vi "Answer.vi"(10 "Accident Number":i32, 11 "NxN":i32) -> (3 "Map":i32[][](array[numeric]))   [LabVIEW 2015]
panel:
  # "地圖"
  # "輸入地圖尺寸"
  # "狀況數量"
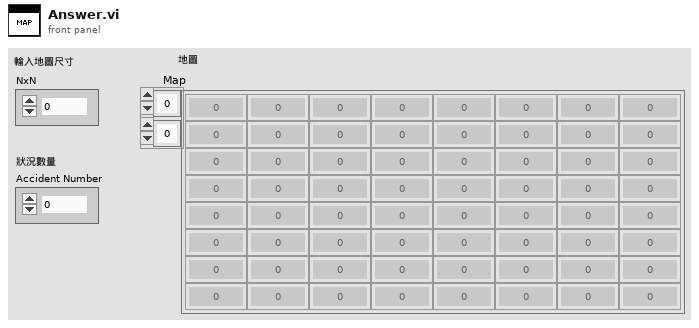
[diagram p1: front panel]
types:
  T1 = typedef "Accident Position.ctl" = cluster{"row":i32, "col":i32}
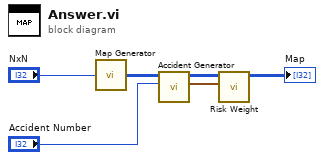
[diagram p0: block diagram]
diagram:
  n1 = call "Map Generator.vi"("NxN"="NxN") -> ("Map"=w5:i32[][])
  n2 = call "Accident Generator.vi"("Accident Number"="Accident Number", "Map"=w5) -> ("Accident Position"=w2:T1[], "Map Out"=w3:i32[][])  [unwired: 8 in]
  n3 = call "Risk Weight.vi"("Accident Position"=w2, "Map"=w3) -> ("Map Out"=→"Map":i32[][])  [unwired: 9 in]
